vi "TestTempDiode.vi"   [LabVIEW 2009]
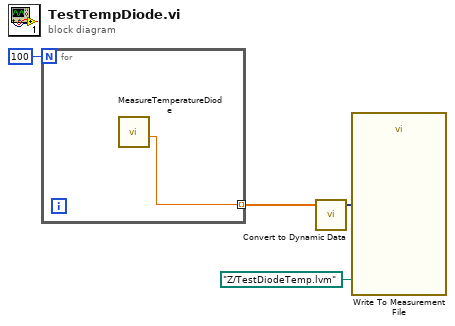
[diagram p0: block diagram]
diagram:
  n1 = for {
    N: 100 -> [_]
    tunnel: [w5] -> w4 mode=indexing
    n2 = call "MeasureTemperatureDiode.vi"() -> ("Celcius"=w5:dbl)  [unwired: 8 in, 3 out]
  }
  n3 = call "Convert to Dynamic Data"("Array"=w4) -> ("Dynamic Data Type"=w3:dynamicdata)  [unwired: 3 in]
  n4 = call "Write To Measurement File"("Signals"=w3, "Filename"=path "Z:/TestDiodeTemp.lvm") -> ()  [unwired: 15 in, 3 out]
